vi "VG_ISOmin.vi"() -> ()   [LabVIEW 2020]
panel:
  out "Iso":dbl
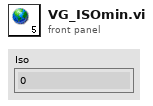
[diagram p1: front panel]
diagram:
